vi "Read Numeric.vi"(11 "Increment Msg in":refnum<class "Increment Msg.lvclass">) -> (2 "Numeric":dbl, 3 "Increment Msg out":refnum<class "Increment Msg.lvclass">)   [LabVIEW 2020, in "Messaging Tests.lvlib" / "Increment Msg.lvclass"]
uses:
  Increment Msg.lvclass
  Increment Msg.lvclass/Increment Msg.ctl
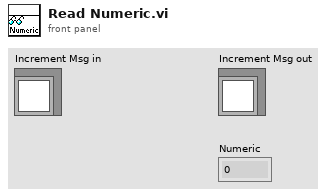
[diagram p1: front panel]
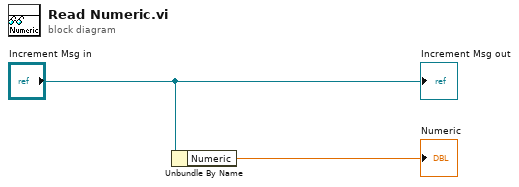
[diagram p0: block diagram]
diagram:
  n1 = Unbundle By Name("Increment Msg in") -> ("Numeric"=→"Numeric":dbl)
  "Increment Msg out" <- "Increment Msg in"
